vi "FeederControl.vi"(5 "Target RPM":dbl, 7 "RPM":dbl, 8 "Buttons":bool[](array[boolean]), 9 "Axes":dbl[](array[numeric])) -> (1 "Output":dbl, 2 "Control Mode":T1)   [LabVIEW 2016]
doc: "This VI mannages the feeder based on the speed and target speed of the shooter. When the user presses the right trigger fully, the feeder will turn on after the shooter HAS BEEN at speed. The feeder can aslo be turned on by pressing the right button.\n\nCreated by Team 4130 for use in the 2016-2017 FRC season"
uses:
  <vilib>/Rock Robotics/WPI/ThirdParty/CanMotor/TalonSRX/WPI_CANTalonSRX_APIControlMode.ctl
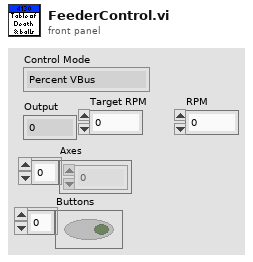
[diagram p1: front panel]
types:
  T1 = typedef "WPI_CANTalonSRX_APIControlMode.ctl" = enum8{"Percent VBus", "Speed", "Position", "Slave", "Unchanged / Invalid", "Voltage Compensation", "Current", "Motion Profile", "Motion Magic"}
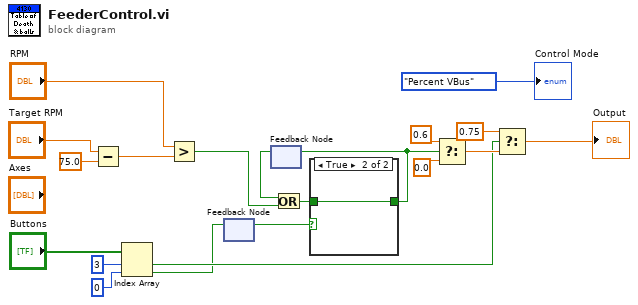
[diagram p0: block diagram]
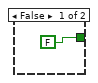
[diagram p2: hidden frame]
diagram:
  n1 = Subtract(x="Target RPM", y=75.0) -> (x-y=w12:dbl)
  n2 = Index Array(array="Buttons", index #1=3 ("index"), index #2=0 ("index")) -> (element #1=w4:bool, element #2=w1:bool)
  n3 = Greater?(x="RPM", y=w12) -> (0:w11:bool)
  n4 = feedback #1() -> (w2:bool)  [unwired: 1 in]
  n5 = feedback-in #1(w1) -> ()
  n6 = feedback #2() -> (w10:bool)  [unwired: 1 in]
  n7 = Or(x=w10, y=w11) -> (x .or. y?=w9:bool)
  n8 = case shown="True" w2 {
    tunnel: [FALSE w22] -> w8
    tunnel: w9 -> [_ w22]
    frame False {
    }
    frame True {
    }
  }
  n9 = feedback-in #2(w8) -> ()
  n10 = Select(t=0.6, s=w8, f=0.0) -> (s? t:f=w7:dbl)
  n11 = Select(t=0.75, s=w4, f=w7) -> (s? t:f=→"Output":dbl)
  "Control Mode" <- WPI_CANTalonSRX_APIControlMode."Percent VBus" ("Control Mode")
